vi "Waveforms.vi"() -> ()   [LabVIEW 2021]
panel:
  out "Digital Waveform Graph":digitalwaveform(graph)
  out "Analog Waveform Graph":waveform(dbl)(graph)
  out "Analog waveform":waveform(dbl)
  out "Digital Waveform":digitalwaveform(waveform)={"t0"=timestamp(0 s since 1904-01-01), "dt"=1.0, "Y"={"transitions"=[], "data"=[]}}
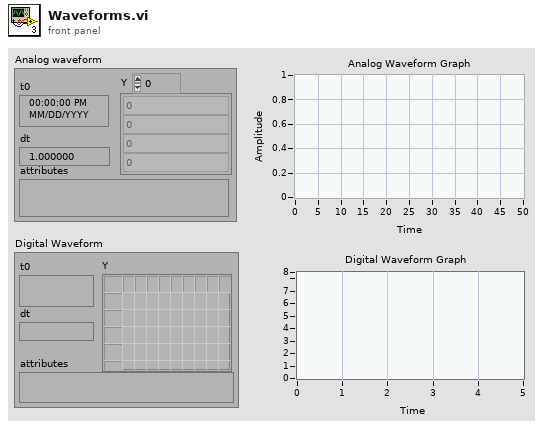
[diagram p1: front panel]
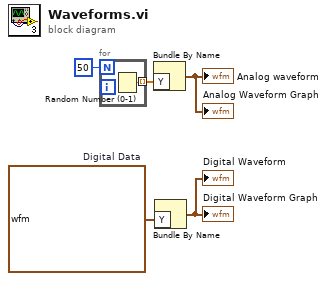
[diagram p0: block diagram]
diagram:
  w3 = digitaldata {"transitions"=[], "data"=[[0, 1, 0, 1, 1, 0, 0, 1], [1, 1, 0, 0, 0, 0, 0, 0], [0, 0, 0, 0, 1, 1, 0, 0], [0, 0, 0, 0, 0, 0, 1, 1], [1, 0, 0, 0, 0, 0, 0, 0]]}  # Digital Data
  n1 = for {
    N: 50 -> [_]
    tunnel: [w6] -> w4 mode=indexing
    n2 = Random Number (0-1)() -> (number: 0 to 1=w6:dbl)
  }
  n3 = Bundle By Name("Y"=w4) -> (→"Analog waveform" →"Analog Waveform Graph":waveform(dbl))  [unwired: 1 in]
  n4 = Bundle By Name("Y"=w3) -> (→"Digital Waveform" →"Digital Waveform Graph":digitalwaveform)  [unwired: 1 in]
